vi "Triggered Tasks-Stop.vi"(8 "error in (no error)":errorcluster, 11 "Logging queue element":T1={"Imaging Protocol"=enum."Live Imaging", "Number of Trials"=0, "Frame Size"=512, "# Averaged frames"=0, "Dwell time (us)"=0.0, "Index of Z-plane"=0, "Timelapse?"=FALSE, "Logging process is active"=FALSE, "Speed logging enabled"=FALSE, "tdms file ref"=refnum, "path"=path "", "Trial Number"=0, "Expected # points acquired"=FALSE, "Manually stopped"=FALSE, "Last trial"=FALSE, "Ch0 data"=[], "Ch1 data"=[], "Image Time"=[], "Continuous Time"=[], "Points acquired"={"Ch0 last trial"=0, "Ch1 last trial"=0, "All trials"=0}, "HW Timings File"=refnum} {"Frame Size" items=["100X100"=100, "128X128"=128, "200X200"=200, "256X256"=256, "512X512"=512, "1024x1024"=1024, "2048x2048"=2048]; "Dwell time (us)" format="%#.6g"}) -> (0 "error out":errorcluster)   [LabVIEW 2017]
uses:
  Typedefs/Logging queue element.ctl
  Typedefs/Imaging Protocols enum.ctl
  Typedefs/Frame Size.ctl
  Typedefs/Acquired points count.ctl
  Typedefs/Read Write Enum.ctl
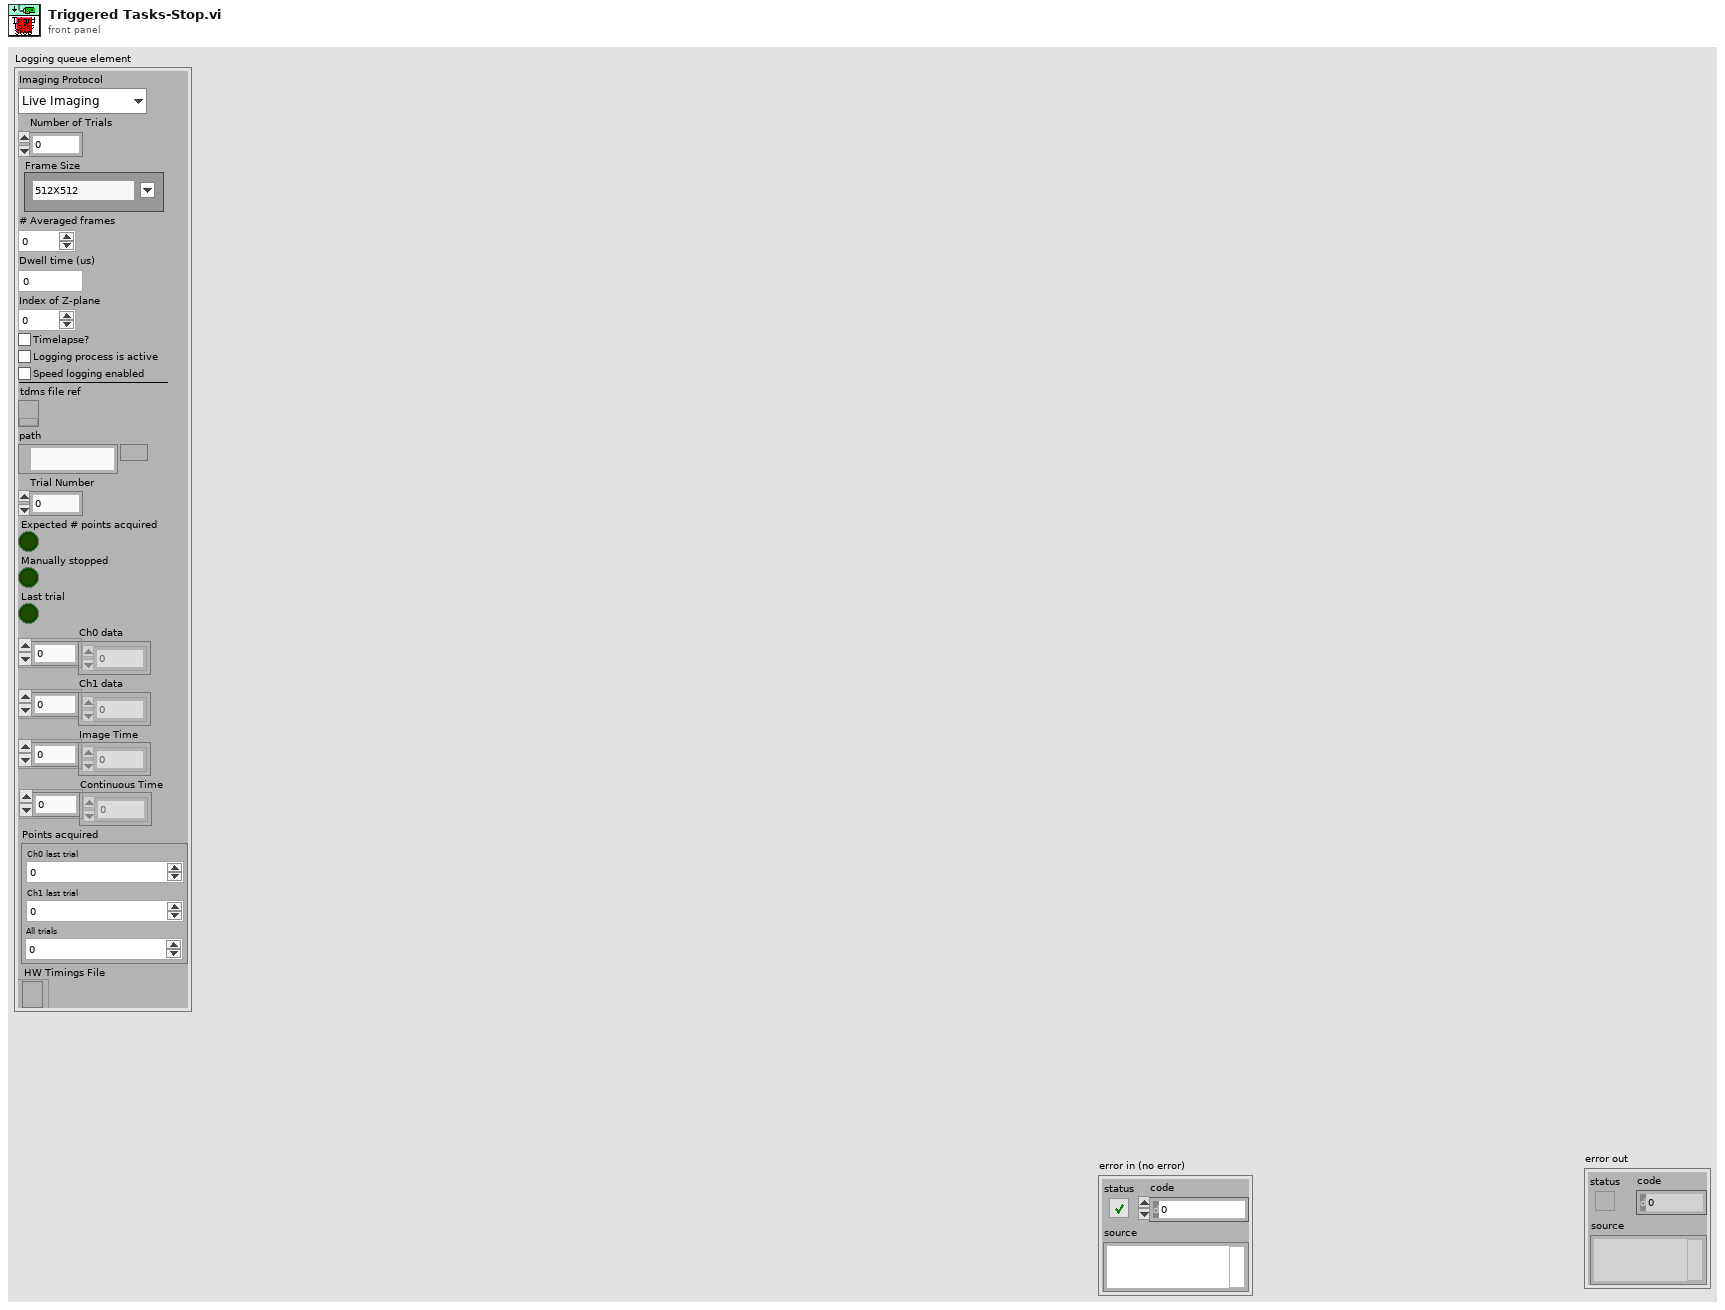
[diagram p1: front panel]
types:
  T1 = typedef "Logging queue element.ctl" = cluster{"Imaging Protocol":T2, "Number of Trials":u16, "Frame Size":T3, "# Averaged frames":u16, "Dwell time (us)":dbl, "Index of Z-plane":i32, "Timelapse?":bool, "Logging process is active":bool, "Speed logging enabled":bool, "tdms file ref":refnum<k34>, "path":path, "Trial Number":i32, "Expected # points acquired":bool, "Manually stopped":bool, "Last trial":bool, "Ch0 data":u32[], "Ch1 data":u32[], "Image Time":u64[], "Continuous Time":u64[], "Points acquired":T4, "HW Timings File":refnum<file>}
  T2 = typedef "Imaging Protocols enum.ctl" = enum16{"AOL Z-Stack", "Motor Z Stack", "Functional Acquisition", "Single Plane Acquisition", "Volume Acquisition", "Live Imaging", "Live Plane Imaging", "Live Volume Imaging"}
  T3 = typedef "Frame Size.ctl" = u16
  T4 = typedef "Acquired points count.ctl" = cluster{"Ch0 last trial":u64, "Ch1 last trial":u64, "All trials":u64}
  T5 = typedef "Read Write Enum.ctl" = enum16{"Read", "Write"}
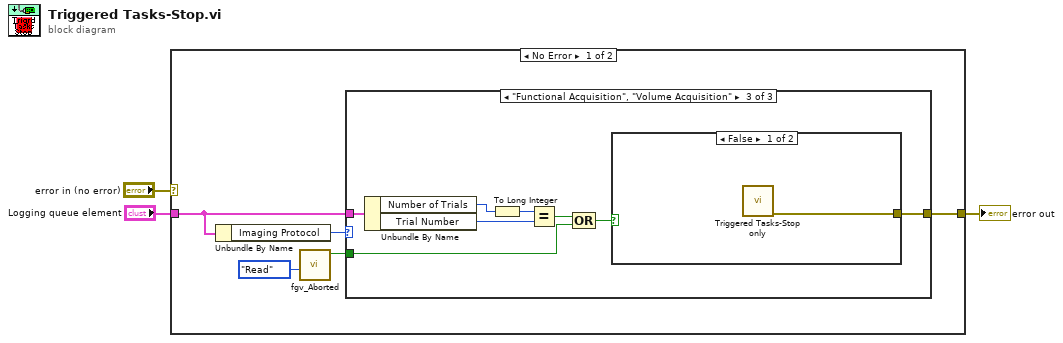
[diagram p0: block diagram]
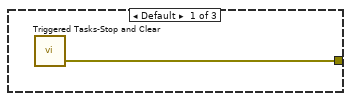
[diagram p2: hidden frame]
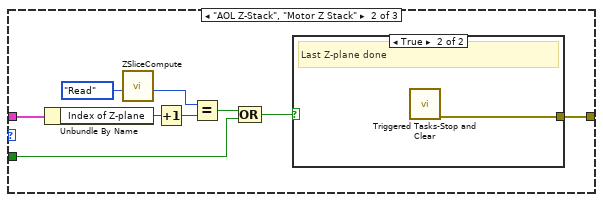
[diagram p3: hidden frame]
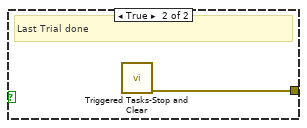
[diagram p5: hidden frame]
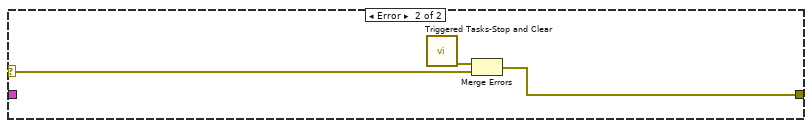
[diagram p6: hidden frame]
diagram:
  n1 = case shown="No Error" "error in (no error)" {
    selector: "error in (no error)" -> [_ w31]
    tunnel: [w8 w30] -> w2
    tunnel: "Logging queue element" -> [w6 _]
    frame No Error {
      n2 = Unbundle By Name(w6) -> ("Imaging Protocol"=w7:T2)
      n3 = call "fgv_Aborted.vi"("Function"=Read_Write_Enum."Read") -> ("Funct Acq Aborted?"=w4:bool)  [unwired: 9 in, 1 out]
      n4 = case shown="\"Functional Acquisition\", \"Volume Acquisition\"" w7 {
        tunnel: w6 -> [_ w18 w27]
        tunnel: [w9 w13 w26] -> w8
        tunnel: w4 -> [_ w10 w20]
        frame Default {
          n5 = call "Triggered Tasks-Stop and Clear.vi"() -> ("error out"=w9:errorcluster)  [unwired: 11 in]
        }
        frame "AOL Z-Stack", "Motor Z Stack" {
          n6 = Unbundle By Name(w18) -> ("Index of Z-plane"=w17:i32)
          n7 = call "ZSliceCompute.vi"("Function"=Read_Write_Enum."Read") -> ("# of Z-planes"=w15:i32)  [unwired: 7 in, 3 out]
          n8 = Increment(x=w17) -> (x+1=w14:i32)
          n9 = Equal?(x=w15, y=w14) -> (x = y?=w12:bool)
          n10 = Compound Arithmetic op=OR(w12, w10) -> (w11:bool)
          n11 = case shown="True" w11 {
            tunnel: [_ w19] -> w13
            frame False {
              # "Not the last plane"
            }
            frame True {
              # "Last Z-plane done"
              n12 = call "Triggered Tasks-Stop and Clear.vi"() -> ("error out"=w19:errorcluster)  [unwired: 11 in]
            }
          }
        }
        frame "Functional Acquisition", "Volume Acquisition" {
          n13 = Unbundle By Name(w27) -> ("Number of Trials"=w24:u16, "Trial Number"=w25:i32)
          n14 = To Long Integer(number=w24) -> (32bit integer=w23:i32)
          n15 = Equal?(x=w23, y=w25) -> (x = y?=w22:bool)
          n16 = Compound Arithmetic op=OR(w22, w20) -> (w21:bool)
          n17 = case shown="False" w21 {
            tunnel: [w28 w29] -> w26
            frame False {
              n18 = call "Triggered Tasks-Stop only.vi"() -> ("error out"=w28:errorcluster)  [unwired: 11 in]
            }
            frame True {
              # "Last Trial done"
              n19 = call "Triggered Tasks-Stop and Clear.vi"() -> ("error out"=w29:errorcluster)  [unwired: 11 in]
            }
          }
        }
      }
    }
    frame Error {
      n20 = call "Triggered Tasks-Stop and Clear.vi"() -> ("error out"=w32:errorcluster)  [unwired: 11 in]
      n21 = Merge Errors(w32, w31) -> (w30:errorcluster)
    }
  }
  "error out" <- w2
